vi "newSetPoint.vi"(8 "error in (no error)":errorcluster, 10 "setTemperature":dbl, 11 "AndorIKonTempController in":refnum<class "AndorIKonTempController.lvclass">) -> (0 "error out":errorcluster, 3 "AndorIKonTempController out":refnum<class "AndorIKonTempController.lvclass">)   [LabVIEW 2011, in "Hardware.lvlib" / "Channels.lvlib" / "AndorIKonTempController.lvclass"]
doc: "Sets a new set point temperature of the Andor camera."
uses:
  AndorIKonTempController.lvclass
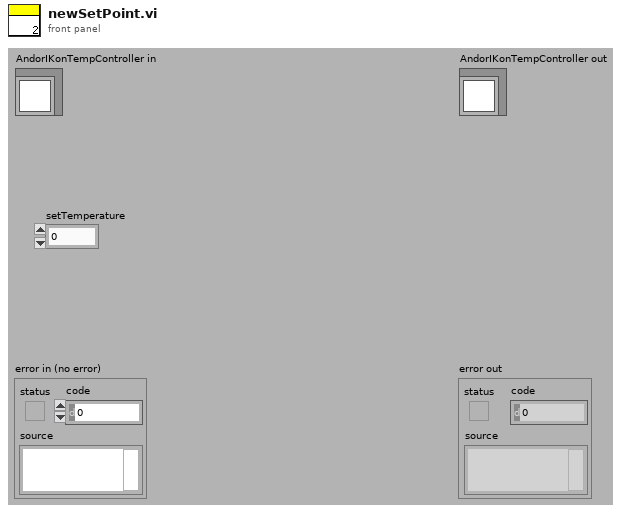
[diagram p1: front panel]
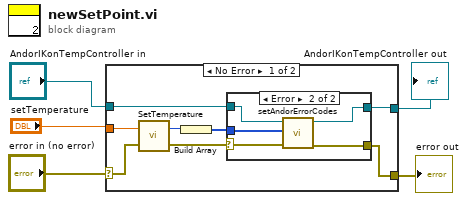
[diagram p0: block diagram]
diagram:
  n1 = case shown="No Error" "error in (no error)" {
    selector: "error in (no error)" -> [w12 w21]
    tunnel: [w6 w21] -> w4
    tunnel: [w8 w22] -> w2
    tunnel: "AndorIKonTempController in" -> [w9 w22]
    tunnel: "setTemperature" -> [w13 _]
    frame No Error {
      n2 = call <userlib>:"SetTemperature.vi"("error in (no error)"=w12, "temperature"=w13) -> ("error out"=w7:errorcluster, "DLL error code"=w11:u32)
      n3 = Build Array(w11) -> (w10:u32[])
      n4 = case shown="Error" w7 {
        selector: w7 -> [w15 w18]
        tunnel: [w15 w17] -> w6
        tunnel: w10 -> [_ w20]
        tunnel: w9 -> [w14 w19]
        tunnel: [w14 w16] -> w8
        frame No Error {
        }
        frame Error {
          n5 = call-dynamic "setAndorErrorCodes.vi"("error in (no error)"=w18, "Andor Error Codes"=w20, "AndorIKonTempController.lvclass in"=w19) -> ("error out"=w17:errorcluster, "AndorIKonTempController.lvclass out"=w16:refnum<class "AndorIKonTempController.lvclass">)  [unwired: 7 in]
        }
      }
    }
    frame Error {
    }
  }
  "error out" <- w4
  "AndorIKonTempController out" <- w2
